vi "filecount.vi"(11 "Path":path) -> (3 "file count string":string)   [LabVIEW 2015]
uses:
  <vilib>/Utility/file.llb/Read From Spreadsheet File (DBL).vi
  <vilib>/Utility/file.llb/Write To Spreadsheet File (DBL).vi
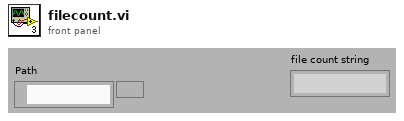
[diagram p1: front panel]
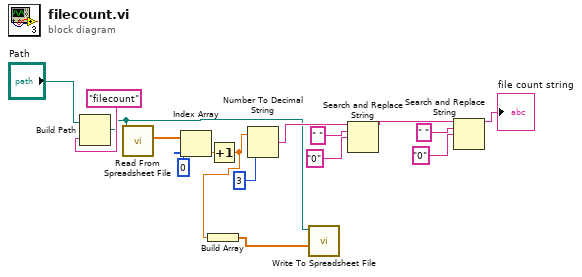
[diagram p0: block diagram]
diagram:
  n1 = Build Path(base path="Path", name or relative path="filecount") -> (appended path=w1:path)
  n2 = call-poly <vilib>:"Read From Spreadsheet File.vi"("file path (dialog if empty)"=w1) -> ("first row"=w15:dbl[])  [unwired: 3 in, 7 out]
  n3 = Index Array(array=w15, index=0) -> (element=w10:dbl)
  n4 = Increment(x=w10) -> (x+1=w3:dbl)
  n5 = Build Array(w3) -> (w2:dbl[])
  n6 = Number To Decimal String(number=w3, width (-)=3) -> (decimal integer string=w11:string)
  n7 = call-poly <vilib>:"Write To Spreadsheet File.vi"("1D data"=w2, "file path (dialog if empty)"=w1) -> ()  [unwired: 4 in, 3 out]
  n8 = Search and Replace String(input string=w11, search string=" ", replace string="0") -> (result string=w6:string)  [unwired: 2 in, 6 out]
  n9 = Search and Replace String(input string=w6, search string=" ", replace string="0") -> (result string=→"file count string":string)  [unwired: 2 in, 6 out]
